vi "Image shift dialog.vi"(5 "Auto close (s)":u32=120, 6 "Data Entry Limits:Increment":dbl=0.1, 7 "Display Format:Precision":u8=1, 8 "Remaining shift (um)":sgl step=0.1 format="%.3g", 9 "Image shift":sgl caption="X shift (nm/image)" step=0.1 format="%.1g", 10 "Caption.Text":string) -> (1 "Image shift (nm/image)":sgl format="%.1g", 2 "Remaining shift frames":u32=1)   [LabVIEW 2018]
panel:
  out "Windows close (s)":u32 caption="Window closes in"
  in  "Done":bool
  # "s"
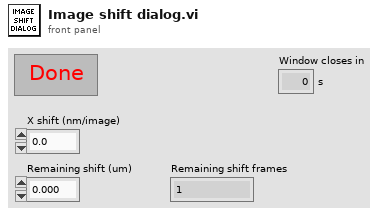
[diagram p1: front panel]
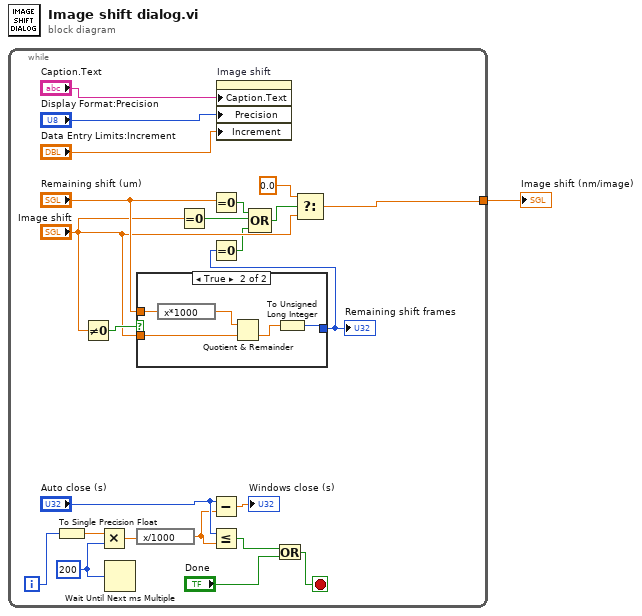
[diagram p0: block diagram]
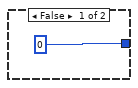
[diagram p2: hidden frame]
diagram:
  n1 = while {
    tunnel: [w10] -> w1
    i -> [w23]
    stop <- w21 stop-if-true
    w24 = u32 200 ("millisecond multiple")
    n2 = To Single Precision Float(number=w23) -> (single precision float=w15:sgl)
    n3 = Not Equal To 0?(x="Image shift") -> (x != 0?=w11:bool)
    n4 = Multiply(x=w15, y=w24) -> (x*y=w20:sgl)
    n5 = Wait Until Next ms Multiple(millisecond multiple=w24) -> ()  [unwired: 1 out]
    n6 = case shown="True" w11 {
      tunnel: "Remaining shift (um)" -> [_ w30]
      tunnel: "Image shift" -> [_ w29]
      tunnel: [u16 0 w26] -> w2
      frame False {
      }
      frame True {
        n7 = expression code="x*1000"(w30) -> (w28:sgl)
        n8 = Quotient & Remainder(x=w28, y=w29) -> (floor(x/y)=w27:sgl)  [unwired: 1 out]
        n9 = To Unsigned Long Integer(number=w27) -> (unsigned 32bit integer=w26:u32)
      }
    }
    "Remaining shift frames" <- w2
    n10 = expression code="x/1000"(w20) -> (w17:sgl)
    n11 = Equal To 0?(x="Image shift") -> (x = 0?=w4:bool)
    n12 = Equal To 0?(x="Remaining shift (um)") -> (x = 0?=w5:bool)
    n13 = Equal To 0?(x=w2) -> (x = 0?=w3:bool)
    n14 = Subtract(x="Auto close (s)", y=w17) -> (x-y=→"Windows close (s)":sgl)
    n15 = Less Or Equal?(x="Auto close (s)", y=w17) -> (x <= y?=w16:bool)
    n16 = property on="Image shift" class="DigNum (strict)"("Caption.Text"="Caption.Text", "Precision"="Display Format:Precision", "Increment"="Data Entry Limits:Increment") -> ()  [unwired: 2 in, 2 out]
    n17 = Compound Arithmetic op=OR(w5, w4, w3) -> (w6:bool)
    n18 = Or(x=w16, y="Done") -> (x .or. y?=w21:bool)
    n19 = Select(t=sgl 0.0 ("Image shift"), s=w6, f="Image shift") -> (s? t:f=w10:sgl)
  }
  "Image shift (nm/image)" <- w1
